vi "7.3.-SubVI Centroide Virtual.vi"(11 "Array 3":path[](array[path])) -> (3 "Array 2":dbl[][](array[numeric]))   [LabVIEW 2020]
panel:
  # "Visión Artificial - Realidad Virtual - Cálculo Centroide\nDiego Cervantes Rodríguez\ndicer0.com"
  # "El Array 3 indica las direcciones de las imágenes izquierda y derecha las cuales se descomponen en forma matricial para poder analizar los colores distintos de cada objeto."
  # "La columna 1 indica los centroides Xi y Xd del primer objeto, la columna 2 las mismas columnas del segundo objeto y así hasta llegar al último objeto."
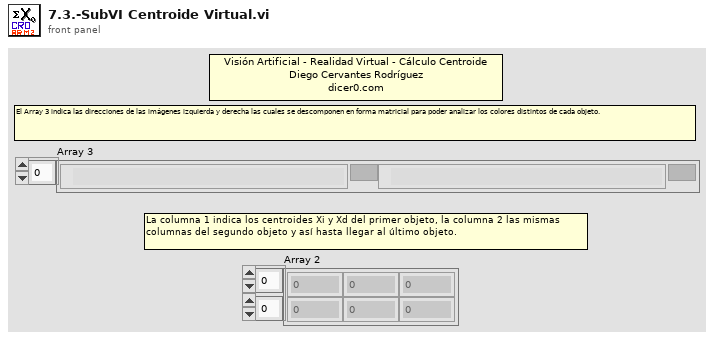
[diagram p1: front panel]
types:
  T1 = typedef "imagedata.ctl" = cluster{"image type":i32, "image depth":i32, "image":u8[], "mask":u8[], "colors":u32[], "Rectangle":cluster{"left":i16, "top":i16, "right":i16, "bottom":i16}}
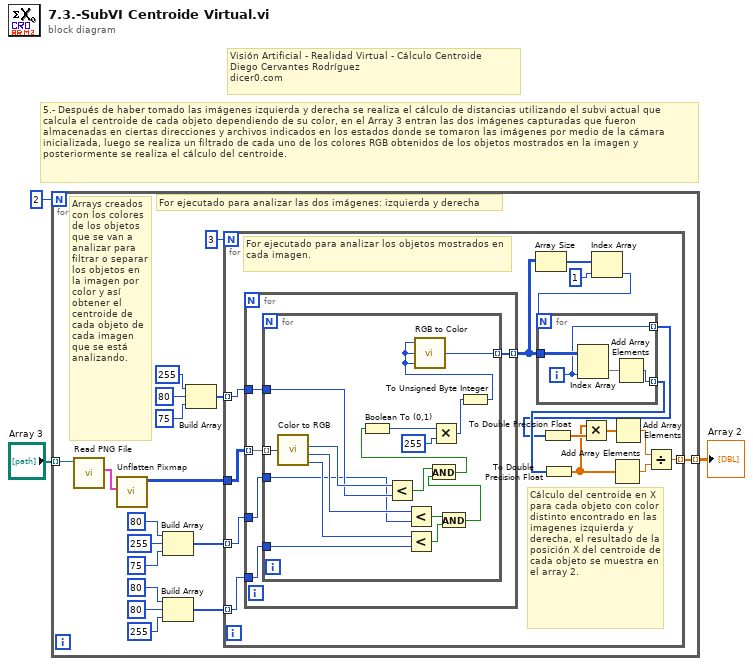
[diagram p0: block diagram]
diagram:
  # "Visión Artificial - Realidad Virtual - Cálculo Centroide\nDiego Cervantes Rodríguez\ndicer0.com"
  # "5.- Después de haber tomado las imágenes izquierda y derecha se realiza el cálculo de distancias utilizando el subvi actual que calcula el centroide de cada objeto dependiendo de su color, en el Array 3 entran las dos imágenes capturadas que fueron almacenadas en ciertas direcciones y archivos indicados en los estados donde se tomaron las imágenes por medio de la cámara inicializada, luego se realiza un filtrado de cada uno de los colores RGB obtenidos de los objetos mostrados en la imagen y posteriormente se realiza el cálculo del centroide."
  n1 = for {
    N: 2 -> [_]
    tunnel: "Array 3" -> [w19] mode=indexing
    tunnel: [w4] -> w3 mode=indexing
    # "Arrays creados con los colores de los objetos que se van a analizar para filtrar o separar los objetos en la imagen por color y así obtener el centroide de cada objeto de cada imagen que se está analizando."
    # "For ejecutado para analizar las dos imágenes: izquierda y derecha"
    n2 = call <vilib>:"Read PNG File.vi"("path to PNG file"=w19) -> ("image data"=w18:T1)  [unwired: 8 in, 2 out]
    n3 = call <vilib>:"Unflatten Pixmap.vi"("image data"=w18) -> ("24-bit pixmap"=w20:u32[][])  [unwired: 4 in, 6 out]
    n4 = Build Array "Build Array"(u8 80 ("y"), u8 255 ("y"), u8 75 ("y")) -> (w6:u8[])
    n5 = Build Array(u8 80 ("y"), u8 80 ("y"), u8 255 ("y")) -> (w5:u8[])
    n6 = Build Array(u8 255 ("y"), u8 80 ("y"), u8 75 ("y")) -> (w13:u8[])
    n7 = for {
      N: 3 -> [_]
      tunnel: w20 -> [w35]
      tunnel: w13 -> [w24] mode=indexing
      tunnel: w6 -> [w23] mode=indexing
      tunnel: w5 -> [w22] mode=indexing
      tunnel: [w21] -> w4 mode=indexing
      # "Cálculo del centroide en X para cada objeto con color distinto encontrado en las imagenes izquierda y derecha, el resultado de la posición X del centroide de cada objeto se muestra en el array 2."
      # "For ejecutado para analizar los objetos mostrados en cada imagen."
      n8 = for {
        tunnel: w35 -> [w45] mode=indexing
        tunnel: [w44] -> w25 mode=indexing
        tunnel: w24 -> [w41]
        tunnel: w23 -> [w42]
        tunnel: w22 -> [w43]
        n9 = for {
          tunnel: w45 -> [w62] mode=indexing
          tunnel: [w61] -> w44 mode=indexing
          tunnel: w43 -> [w46]
          tunnel: w42 -> [w47]
          tunnel: w41 -> [w48]
          n10 = call <vilib>:"Color to RGB.vi"("Color"=w62) -> ("R"=w57:u8, "G"=w55:u8, "B"=w49:u8)  [unwired: 1 out]
          n11 = Less?(x=w57, y=w48) -> (x < y?=w51:bool)
          n12 = Less?(x=w55, y=w47) -> (x < y?=w53:bool)
          n13 = Less?(x=w49, y=w46) -> (x < y?=w54:bool)
          n14 = And(x=w53, y=w54) -> (x .and. y?=w52:bool)
          n15 = And(x=w51, y=w52) -> (x .and. y?=w50:bool)
          n16 = Boolean To (0,1)(Boolean=w50) -> (0, 1=w60:i16)
          n17 = Multiply(x=w60, y=i16 255) -> (x*y=w59:i16)
          n18 = To Unsigned Byte Integer(number=w59) -> (unsigned 8bit integer=w56:u8)
          n19 = call <vilib>:"RGB to Color.vi"("B"=w56, "G"=w56, "R"=w56) -> ("Color"=w61:u32)
        }
      }
      n20 = Array Size(array=w25) -> (size(s)=w26:i32[])
      n21 = Index Array "Index Array"(array=w26, index=1) -> (element=w28:i32)
      n22 = for {
        N: w28 -> [_]
        tunnel: w25 -> [w40]
        tunnel: [w38] -> w33 mode=indexing
        tunnel: [w37] -> w32 mode=indexing
        i -> [w37]
        n23 = Index Array "Index Array"(array=w40, index (col)=w37) -> (element=w39:u32[])  [unwired: 1 in]
        n24 = Add Array Elements(numeric array=w39) -> (sum=w38:u32)
      }
      n25 = To Double Precision Float(number=w32) -> (double precision float=w36:dbl[])
      n26 = To Double Precision Float(number=w33) -> (double precision float=w34:dbl[])
      n27 = Multiply(x=w34, y=w36) -> (x*y=w30:dbl[])
      n28 = Add Array Elements(numeric array=w34) -> (sum=w31:dbl)
      n29 = Add Array Elements(numeric array=w30) -> (sum=w29:dbl)
      n30 = Divide(x=w29, y=w31) -> (x/y=w21:dbl)
    }
  }
  "Array 2" <- w3
